vi "Calculate Gain and Phase.vi"(1 "Response":T1[](array[typedef]) {"Freq" format="%#.2f"; "Offset" format="%.3f"; "Gain" format="%.2f"; "Phase" format="%.1f"}, 2 "Stimulus":T1[](array[typedef]) {"Freq" format="%#.2f"; "Offset" format="%.3f"; "Gain" format="%.2f"; "Phase" format="%.1f"}) -> (0 "Gain and Phase out":T2 {"Phase SD" format="%.1f"; "Phase" format="%.1f"; "Gain SD" format="%.2f"; "Gain" format="%.2f"})   [LabVIEW 2016, in "Sinusoidal Fit.lvclass"]
uses:
  Sinusoidal Fit.lvclass
  gain and phase/Typedef - Gain and Phase.ctl
  gain and phase/Typedef - Sinusoidal Fit Coefficients.ctl
  comm/nan operations/nan operations.lvlib
panel:
  # "Gain:"
  # "+/-"
  # "Phase:"
  # "+/-"
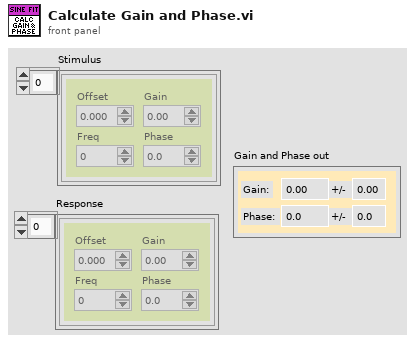
[diagram p1: front panel]
types:
  T1 = typedef "Typedef - Sinusoidal Fit Coefficients.ctl" = cluster{"Offset":dbl, "Gain":dbl, "Phase":dbl, "Freq":dbl}
  T2 = typedef "Typedef - Gain and Phase.ctl" = cluster{"Gain":dbl, "Gain SD":dbl, "Phase":dbl, "Phase SD":dbl}
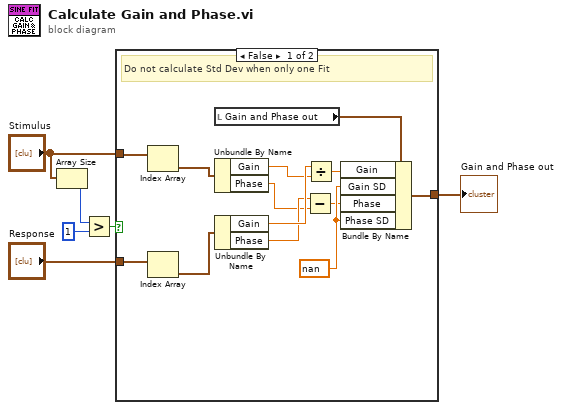
[diagram p0: block diagram]
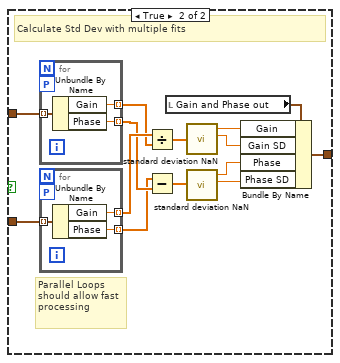
[diagram p2: hidden frame]
diagram:
  n1 = Array Size(array="Stimulus") -> (size(s)=w2:i32)
  n2 = Greater?(x=w2, y=1) -> (0:w3:bool)
  n3 = case shown="False" w3 {
    tunnel: "Stimulus" -> [w18 w33]
    tunnel: "Response" -> [w19 w32]
    tunnel: [w14 w28] -> w5
    frame False {
      w17 = nan
      # "Do not calculate Std Dev when only one Fit"
      n4 = Index Array(array=w18) -> (element=w13:T1)  [unwired: 1 in]
      n5 = Index Array(array=w19) -> (element=w12:T1)  [unwired: 1 in]
      n6 = local read "Gain and Phase out"() -> (w11:T2)
      n7 = Unbundle By Name(w13) -> ("Gain"=w9:dbl, "Phase"=w7:dbl)
      n8 = Unbundle By Name(w12) -> ("Gain"=w10:dbl, "Phase"=w8:dbl)
      n9 = Subtract(x=w8, y=w7) -> (x-y=w16:dbl)
      n10 = Divide(x=w10, y=w9) -> (x/y=w15:dbl)
      n11 = Bundle By Name(cluster=w11, "Gain"=w15, "Gain SD"=w17, "Phase"=w16, "Phase SD"=w17) -> (w14:T2)
    }
    frame True {
      # "Parallel Loops should allow fast processing"
      # "Calculate Std Dev with multiple fits"
      n12 = for {
        workers-P: _ -> [_]
        tunnel: w33 -> [w39] mode=indexing
        tunnel: [w38] -> w22 mode=indexing
        tunnel: [w37] -> w21 mode=indexing
        n13 = Unbundle By Name(w39) -> ("Gain"=w38:dbl, "Phase"=w37:dbl)
      }
      n14 = for {
        workers-P: _ -> [_]
        tunnel: w32 -> [w36] mode=indexing
        tunnel: [w35] -> w23 mode=indexing
        tunnel: [w34] -> w20 mode=indexing
        n15 = Unbundle By Name(w36) -> ("Gain"=w35:dbl, "Phase"=w34:dbl)
      }
      n16 = Divide(x=w23, y=w22) -> (x/y=w31:dbl[])
      n17 = Subtract(x=w20, y=w21) -> (x-y=w30:dbl[])
      n18 = local read "Gain and Phase out"() -> (w29:T2)
      n19 = call "standard deviation NaN.vi"("Array"=w31) -> ("standard deviation"=w26:dbl, "mean"=w27:dbl)  [unwired: 2 in, 1 out]
      n20 = call "standard deviation NaN.vi"("Array"=w30) -> ("standard deviation"=w24:dbl, "mean"=w25:dbl)  [unwired: 2 in, 1 out]
      n21 = Bundle By Name(cluster=w29, "Gain"=w27, "Gain SD"=w26, "Phase"=w25, "Phase SD"=w24) -> (w28:T2)
    }
  }
  "Gain and Phase out" <- w5
